vi "Table, Delete All Values.vi"(8 "error in":errorcluster, 11 "Tbl Refnum":refnum<vi>) -> (0 "error out":errorcluster, 3 "Tbl Refnum dup":refnum<vi>)   [LabVIEW 2010]
doc: "Shows all table rows plus an empty row.\nSince all rows are displayed, the vertical scrollbar is hidden."
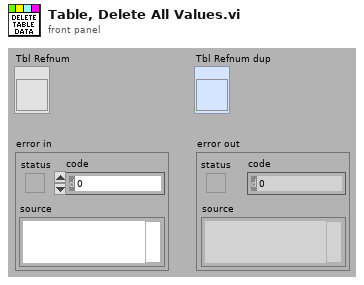
[diagram p1: front panel]
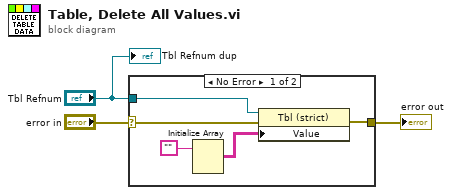
[diagram p0: block diagram]
diagram:
  n1 = case shown="No Error" "error in" {
    selector: "error in" -> [w7 w9]
    tunnel: [w6 w9] -> w3
    tunnel: "Tbl Refnum" -> [w8 _]
    frame No Error {
      n2 = Initialize Array("") -> (w4:string[][])  [unwired: 2 in]
      n3 = property class="Tbl (strict)"(reference=w8, error in=w7, "Value"=w4) -> (error out=w6:errorcluster)  [unwired: 1 out]
    }
    frame Error {
    }
  }
  "error out" <- w3
  "Tbl Refnum dup" <- "Tbl Refnum"
